vi "Nano-Drive Information.vi"(0 "Handle":i32) -> (8 "ADC resolution (bits)":i16, 10 "DAC resolution (bits)":i16, 12 "Product ID (in hex)":string, 13 "Serial #":i32, 14 "Firmware Version":i16, 15 "DAC Freq (ms)":dbl format="%.4f", 16 "Firmware Profile":i16, 17 "ADC Freq (ms)":dbl format="%.4f", 18 "Dll Version":i16, 19 "Dll Revision":i16, 20 "X axis":bool, 21 "Y axis":bool, 22 "Z axis":bool, 23 "Aux axis":bool, 24 "X Calibration":dbl caption="Calibration (um)" format="%.3f", 25 "Y Calibration":dbl format="%.3f", 26 "Z Calibration":dbl format="%.3f", 27 "Aux Calibration":dbl format="%.3f")   [LabVIEW 2012]
uses:
  Madlib.dll
panel:
  # "This example VI provides access to (and demonstrates how to access)\n important device information."
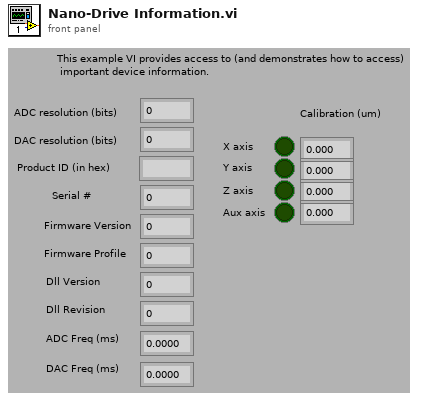
[diagram p1: front panel]
types:
  T1 = cluster{u8, u8, u8, u8, u8, u8, u8, u8, u8, u8, u8}
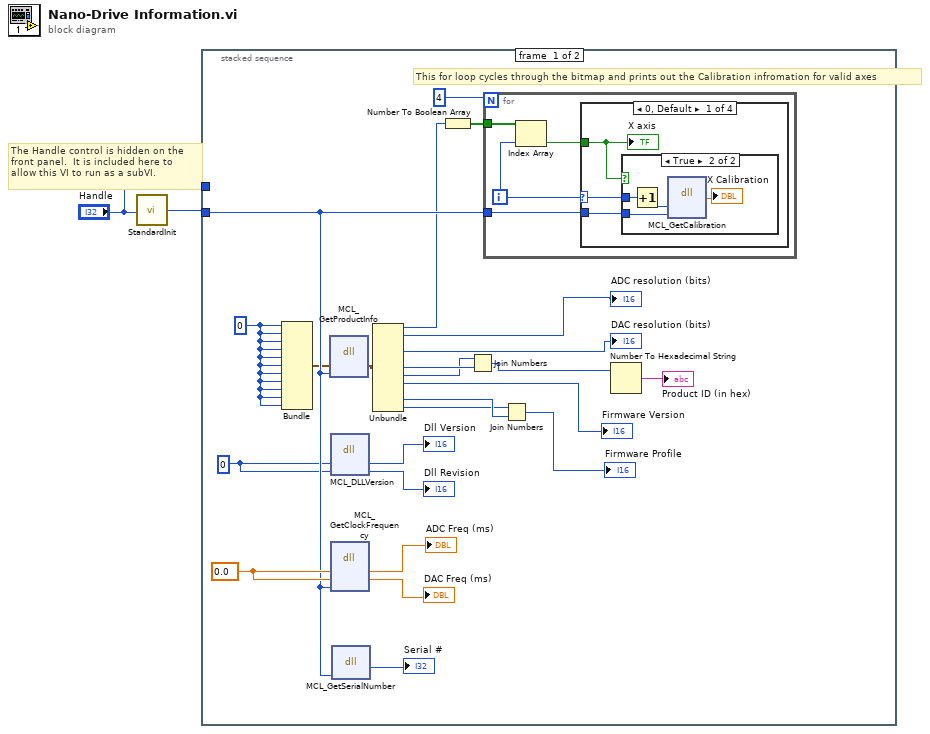
[diagram p0: block diagram]
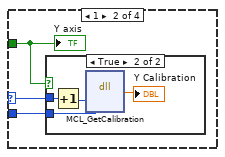
[diagram p3: hidden frame]
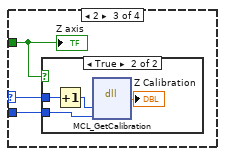
[diagram p5: hidden frame]
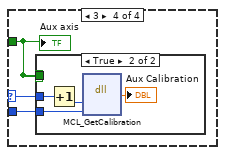
[diagram p7: hidden frame]
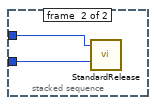
[diagram p9: hidden frame]
diagram:
  # "The Handle control is hidden on the\nfront panel.  It is included here to\nallow this VI to run as a subVI."
  n1 = call "StandardInit.vi"("Incoming Handle"="Handle") -> ("Outgoing Handle"=w2:i32)
  n2 = stacked-sequence {
    tunnel: w2 -> [w17 w60]
    tunnel: "Handle" -> [_ w59]
    frame #0 {
      w16 = i16 0
      w23 = 0.0
      w13 = u8 0
      # "This for loop cycles through the bitmap and prints out the Calibration infromation for valid axes"
      n3 = Bundle(w13, w13, w13, w13, w13, w13, w13, w13, w13, w13, w13) -> (w15:T1)  [unwired: 1 out]
      n4 = dll-call lib="C:/Users/Labview/Desktop/Labview Examples/MADLib.dll" fn="MCL_GetProductInfo"(w15, "handle"=w17) -> (w14:T1)  [unwired: 5 in, 2 out]
      n5 = dll-call lib="C:/Users/Labview/Desktop/Labview Examples/MADLib.dll" fn="MCL_DLLVersion"("version"=w16, "revision"=w16) -> ("version"=→"Dll Version":i16, "revision"=→"Dll Revision":i16)  [unwired: 4 in, 2 out]
      n6 = dll-call lib="C:/Users/Labview/Desktop/Labview Examples/MADLib.dll" fn="MCL_GetClockFrequency"("ADC freq"=w23, "DAC freq"=w23, "handle"=w17) -> ("ADC freq"=→"ADC Freq (ms)":dbl, "DAC freq"=→"DAC Freq (ms)":dbl)  [unwired: 5 in, 2 out]
      n7 = dll-call lib="C:/Users/Labview/Desktop/Labview Examples/MADLib.dll" fn="MCL_GetSerialNumber"("handle"=w17) -> (→"Serial #":i32)  [unwired: 4 in, 2 out]
      n8 = Unbundle(w14) -> (w12:u8, →"ADC resolution (bits)":u8, →"DAC resolution (bits)":u8, w9:u8, w8:u8, →"Firmware Version":u8, w5:u8, w4:u8)  [unwired: 3 out]
      n9 = Number To Boolean Array(number=w12) -> (Boolean array=w20:bool[])
      n10 = Join Numbers(hi=w8, lo=w9) -> ((hi.lo)=w7:u16)
      n11 = for {
        N: 4 -> [_]
        tunnel: w20 -> [w30]
        tunnel: w17 -> [w27]
        i -> [w29]
        n12 = Index Array(array=w30, index=w29) -> (element=w28:bool)
        n13 = case shown="0, Default" w29 {
          selector: w29 -> [w33 w40 w47 w54]
          tunnel: w28 -> [w32 w39 w46 w53]
          tunnel: w27 -> [w31 w38 w45 w52]
          frame 0, Default {
            n14 = case shown="True" w32 {
              tunnel: w33 -> [_ w37]
              tunnel: w31 -> [_ w34]
              frame False {
              }
              frame True {
                n15 = Increment(x=w37) -> (x+1=w35:i32)
                n16 = dll-call lib="C:/Users/Labview/Desktop/Labview Examples/MADLib.dll" fn="MCL_GetCalibration"("axis"=w35, "handle"=w34) -> (→"X Calibration":dbl)  [unwired: 5 in, 2 out]
              }
            }
            "X axis" <- w32
          }
          frame 1 {
            n17 = case shown="True" w39 {
              tunnel: w40 -> [_ w44]
              tunnel: w38 -> [_ w42]
              frame False {
              }
              frame True {
                n18 = Increment(x=w44) -> (x+1=w43:i32)
                n19 = dll-call lib="C:/Users/Labview/Desktop/Labview Examples/MADLib.dll" fn="MCL_GetCalibration"("axis"=w43, "handle"=w42) -> (→"Y Calibration":dbl)  [unwired: 5 in, 2 out]
              }
            }
            "Y axis" <- w39
          }
          frame 2 {
            n20 = case shown="True" w46 {
              tunnel: w47 -> [_ w51]
              tunnel: w45 -> [_ w49]
              frame False {
              }
              frame True {
                n21 = Increment(x=w51) -> (x+1=w48:i32)
                n22 = dll-call lib="C:/Users/Labview/Desktop/Labview Examples/MADLib.dll" fn="MCL_GetCalibration"("axis"=w48, "handle"=w49) -> (→"Z Calibration":dbl)  [unwired: 5 in, 2 out]
              }
            }
            "Z axis" <- w46
          }
          frame 3 {
            n23 = case shown="True" w53 {
              tunnel: w54 -> [_ w58]
              tunnel: w53 -> [_ _]
              tunnel: w52 -> [_ w55]
              frame False {
              }
              frame True {
                n24 = Increment(x=w58) -> (x+1=w56:i32)
                n25 = dll-call lib="C:/Users/Labview/Desktop/Labview Examples/MADLib.dll" fn="MCL_GetCalibration"("axis"=w56, "handle"=w55) -> (→"Aux Calibration":dbl)  [unwired: 5 in, 2 out]
              }
            }
            "Aux axis" <- w53
          }
        }
      }
      n26 = Join Numbers(hi=w4, lo=w5) -> ((hi.lo)=→"Firmware Profile":u16)
      n27 = Number To Hexadecimal String(2:w7) -> (0:→"Product ID (in hex)":string)  [unwired: 1 in]
    }
    frame #1 {
      n28 = call "StandardRelease.vi"("Outgoing Handle"=w60, "Incoming Handle"=w59) -> ()  [unwired: 1 in]
    }
  }
